vi "Write Last Series.vi"(10 "Series":refnum<class "Series.lvclass">, 11 "Result in":refnum<class "Result.lvclass">) -> (3 "Result out":refnum<class "Result.lvclass">)   [LabVIEW 2018, in "InfluxDB Client.lvlib" / "Result.lvclass"]
uses:
  Result.lvclass
  Series/Series.lvclass
  Result.lvclass/Result.ctl
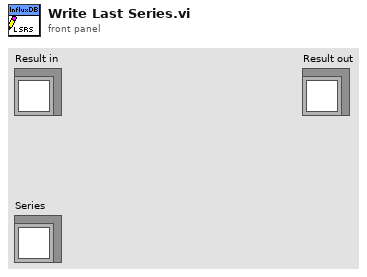
[diagram p1: front panel]
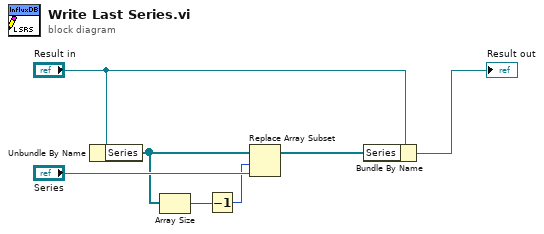
[diagram p0: block diagram]
diagram:
  n1 = Unbundle By Name("Result in") -> ("Series"=w3:refnum<class "Series.lvclass">[])
  n2 = Array Size(array=w3) -> (size(s)=w2:i32)
  n3 = Decrement(x=w2) -> (x-1=w1:i32)
  n4 = Replace Array Subset(array=w3, new element="Series", index=w1) -> (w4:refnum<class "Series.lvclass">[])
  n5 = Bundle By Name(cluster="Result in", "Series"=w4) -> (→"Result out":refnum<class "Result.lvclass">)
